vi "De Jitter Data.vi"(10 "Target Info":dbl[][](array[numeric]) format="%#.1f") -> (2 "Filtered Data":dbl[][](array[numeric]))   [LabVIEW 2025]
panel:
  # "Distance"
  # "Angle"
  # "Tag #"
  # "Yaw"
  # "Pitch"
  # "Roll"
  # "Camera #"
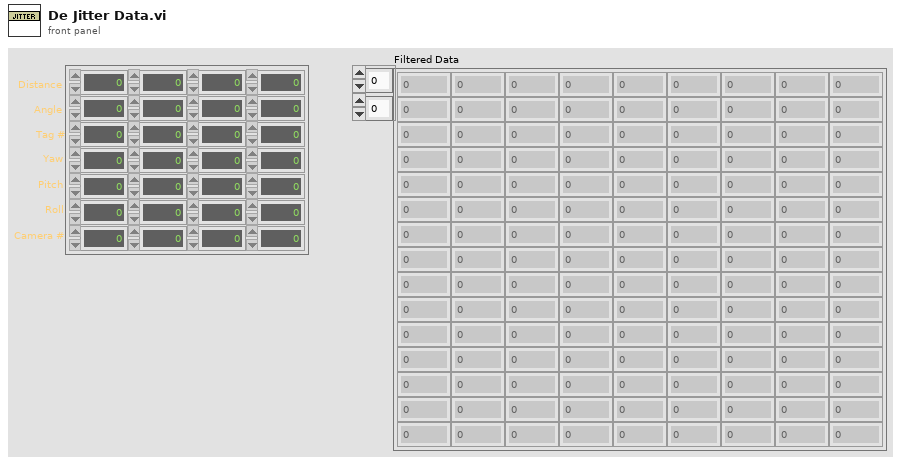
[diagram p1: front panel]
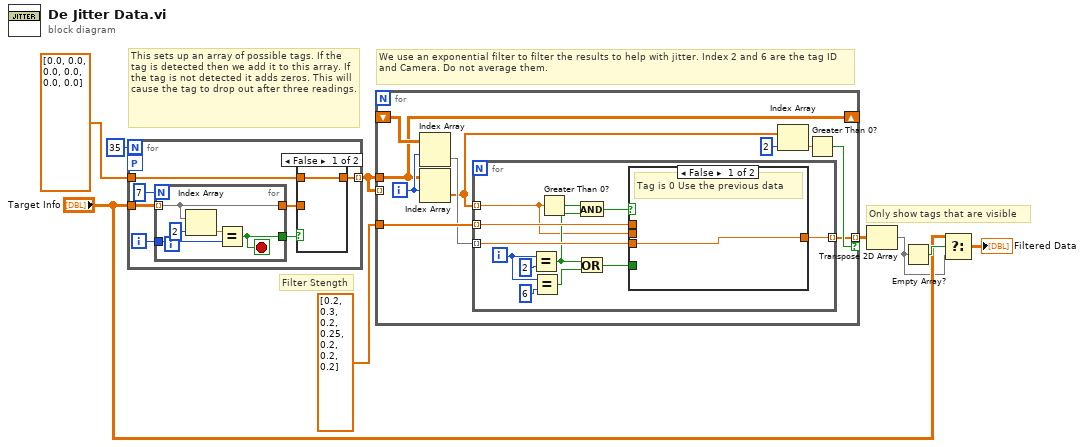
[diagram p0: block diagram]
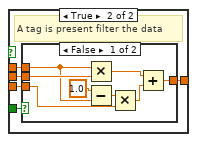
[diagram p2: hidden frame]
diagram:
  # "Filter Stength"
  # "Only show tags that are visible"
  # "We use an exponential filter to filter the results to help with jitter. Index 2 and 6 are the tag ID and Camera. Do not average them."
  # "This sets up an array of possible tags. If the tag is detected then we add it to this array. If the tag is not detected it adds zeros. This will cause the tag to drop out after three readings."
  n1 = for {
    N: 35 -> [_]
    tunnel: dbl[] [0.0, 0.0, 0.0, 0.0, 0.0, 0.0] ("f") -> [w13]
    tunnel: "Target Info" -> [w14]
    tunnel: [w12] -> w6 mode=indexing
    workers-P: _ -> [_]
    i -> [w11]
    n2 = for {
      N: 7 -> [_]
      tunnel: [w18] -> w16
      tunnel: [w19] -> w15
      tunnel: w14 -> [w19] mode=indexing
      tunnel: w11 -> [w20]
      stop <- w18 stop-if-true
      n3 = Index Array(array=w19, index=2) -> (element=w21:dbl)
      n4 = Equal?(x=w21, y=w20) -> (x = y?=w18:bool)
    }
    n5 = case shown="False" w16 {
      tunnel: w15 -> [_ w23]
      tunnel: [w22 w23] -> w12
      tunnel: w13 -> [w22 _]
      frame False {
      }
      frame True {
      }
    }
  }
  n6 = for {
    tunnel: w6 -> [w24]
    shift-right: [w24] -> _
    shift-left: _ -> [w33]
    tunnel: [w31] -> w7 mode=indexing if=w32
    tunnel: w6 -> [_] mode=indexing
    tunnel: dbl[] [0.2, 0.3, 0.2, 0.25, 0.2, 0.2, 0.2] -> [w30]
    i -> [w29]
    n7 = Index Array(array=w33, index (row)=w29) -> (element=w26:dbl[])  [unwired: 1 in]
    n8 = Index Array(array=w24, index (row)=w29) -> (element=w25:dbl[])  [unwired: 1 in]
    n9 = for {
      tunnel: w25 -> [w34] mode=indexing
      tunnel: w26 -> [w45] mode=indexing
      tunnel: [w44] -> w31 mode=indexing
      tunnel: w30 -> [w39] mode=indexing
      i -> [w35]
      n10 = Equal?(x=w35, y=2) -> (x = y?=w37:bool)
      n11 = Equal?(x=w35, y=6) -> (x = y?=w41:bool)
      n12 = Greater Than 0?(x=w34) -> (x > 0?=w36:bool)
      n13 = And(x=w36, y=w37) -> (x .and. y?=w38:bool)
      n14 = Or(x=w37, y=w41) -> (x .or. y?=w40:bool)
      n15 = case shown="False" w38 {
        tunnel: w34 -> [_ w51]
        tunnel: w45 -> [w46 w50]
        tunnel: [w46 w49] -> w44
        tunnel: w40 -> [_ w48]
        tunnel: w39 -> [_ w47]
        frame False {
          # "Tag is 0 Use the previous data"
        }
        frame True {
          # "A tag is present filter the data"
          n16 = case shown="False" w48 {
            tunnel: w51 -> [w59 _]
            tunnel: w50 -> [w56 w60]
            tunnel: [w53 w60] -> w49
            tunnel: w47 -> [w52 _]
            frame False {
              n17 = Multiply(x=w52, y=w59) -> (x*y=w54:dbl)
              n18 = Subtract(x=1.0, y=w52) -> (x-y=w57:dbl)
              n19 = Multiply(x=w57, y=w56) -> (x*y=w55:dbl)
              n20 = Add(x=w54, y=w55) -> (x+y=w53:dbl)
            }
            frame True {
            }
          }
        }
      }
    }
    n21 = Index Array(array=w25, index=2) -> (element=w27:dbl)
    n22 = Greater Than 0?(x=w27) -> (x > 0?=w32:bool)
  }
  n23 = Transpose 2D Array(2D array=w7) -> (transposed array=w1:dbl[][])
  n24 = Empty Array?(array=w1) -> (empty?=w4:bool)
  n25 = Select(t="Target Info", s=w4, f=w1) -> (s? t:f=→"Filtered Data":dbl[][])
